vi "Create XY Plot Histogram.vi"(8 "error in (no error)":errorcluster, 11 "Plot Histogram Call Parameters":T1={"XY Graph Refnum"=refnum, "Mouse Click Coords"={"Horizontal"=2147483647, "Vertical"=2147483647}, "Plot Index"=-1, "Histogram Options"={"Bin Size"=nan, "Bin Number"=0, "Bin Option"=enum."Bin Number", "Min Value"=-inf, "Max Value"=inf, "Filter NaN & Infinite Values"=TRUE, "Frequency Plot"=FALSE, "Align Bins"=FALSE, "Bin Location"=enum."Left", "Project Outside Values"=FALSE, "Max Histogram Size"=100000}} {"Histogram Options"."Max Histogram Size" format="%.0e"}) -> (0 "error out":errorcluster, 1 "Message":string, 3 "Histogram Statistics":dbl[](array[numeric]))   [LabVIEW 2021, in "Histogram Window.lvlib"]
uses:
  Histogram Window.lvlib
  Histogram Call Parameters.ctl
  Graphs/XY Graph/XY Graph Refnum.ctl
  <vilib>/Utility/miscctls.llb/LVPoint32TypeDef.ctl
  Linear Histogram Options.ctl
  Histogram Bin Option.ctl
  Histogram Bin Position.ctl
  Graphs/XY Graph/XY Graph Add-Ons.lvlib
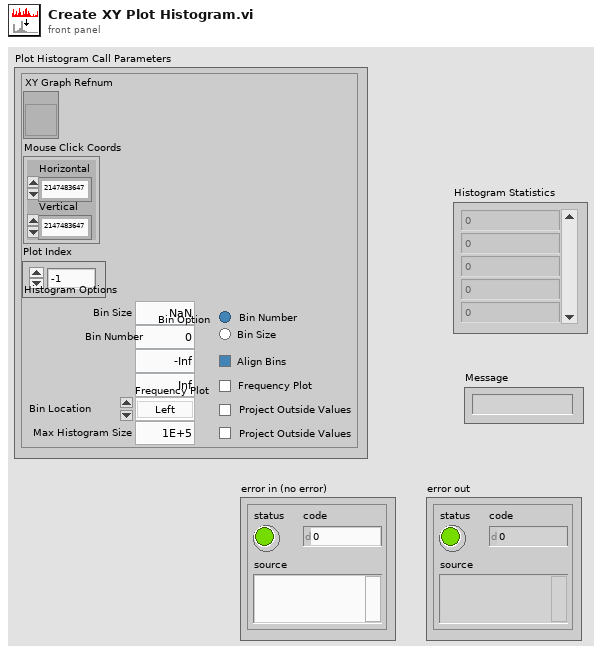
[diagram p1: front panel]
types:
  T1 = typedef "Histogram Window.lvlib/Histogram Call Parameters.ctl" = cluster{"XY Graph Refnum":T2, "Mouse Click Coords":T3, "Plot Index":i32, "Histogram Options":T4}
  T2 = typedef "XY Graph Add-Ons.lvlib/XY Graph Refnum.ctl" = refnum<vi>
  T3 = typedef "LVPoint32TypeDef.ctl" = cluster{"Horizontal":i32, "Vertical":i32}
  T4 = typedef "Histogram Window.lvlib/Linear Histogram Options.ctl" = cluster{"Bin Size":dbl, "Bin Number":i32, "Bin Option":T5, "Min Value":dbl, "Max Value":dbl, "Filter NaN & Infinite Values":bool, "Frequency Plot":bool, "Align Bins":bool, "Bin Location":T6, "Project Outside Values":bool, "Max Histogram Size":i32}
  T5 = typedef "Histogram Window.lvlib/Histogram Bin Option.ctl" = enum32{"Bin Number", "Bin Size"}
  T6 = typedef "Histogram Window.lvlib/Histogram Bin Position.ctl" = enum16{"Left", "Center", "Right"}
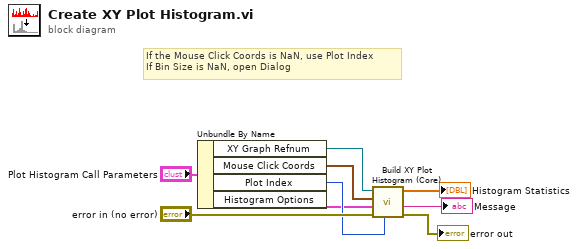
[diagram p0: block diagram]
diagram:
  # "If the Mouse Click Coords is NaN, use Plot Index\nIf Bin Size is NaN, open Dialog"
  n1 = Unbundle By Name("Plot Histogram Call Parameters") -> ("XY Graph Refnum"=w7:T2, "Mouse Click Coords"=w5:T3, "Plot Index"=w4:i32, "Histogram Options"=w2:T4)
  n2 = call "Build XY Plot Histogram (Core).vi"("Plot Index (-1: last)"=w4, "error in (no error)"="error in (no error)", "Histogram Options (Default: dialog)"=w2, "Mouse Click Coords (default: use Plot Index)"=w5, "XYGraph in"=w7) -> ("error out"=→"error out":errorcluster, "Message"=→"Message":string, "Data Statistics"=→"Histogram Statistics":dbl[])  [unwired: 4 in]
